vi "Read Start Sequence Button.vi"(4 "error in":errorcluster) -> (0 "error out":errorcluster, 2 "Start Button Pressed?":bool)   [LabVIEW 2015]
uses:
  <vilib>/DAQmx/read.llb/DAQmx Read (Digital Bool 1Line 1Point).vi
  <vilib>/DAQmx/miscellaneous.llb/DAQmx Fill In Error Info.vi
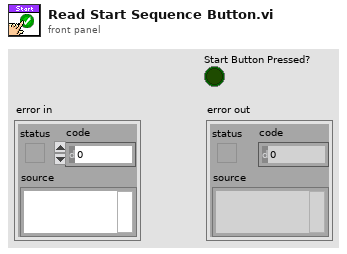
[diagram p1: front panel]
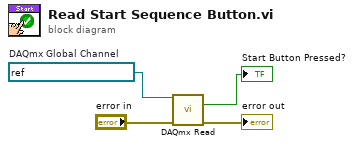
[diagram p0: block diagram]
diagram:
  w4 = refnum<k21> "DI3 Start Sequence"  # DAQmx Global Channel
  n1 = call-poly <vilib>:"DAQmx Read.vi"("task/channels in"=w4, "error in"="error in") -> ("data"=→"Start Button Pressed?":bool, "error out"=→"error out":errorcluster)  [unwired: 11 in, 1 out]
